vi "TIFF Default Strip Size.vi"(8 "error in (no error)":errorcluster, 10 "para1":cluster{}, 11 "para0":cluster{}) -> (0 "error out":errorcluster, 2 "function return":u32, 3 "para0 out":cluster{})   [LabVIEW 2018]
doc: "LIBTIFF_DLL_IMPEXP uint32 TIFFDefaultStripSize(TIFF*, uint32);\nextern uint32 TIFFDefaultStripSize(TIFF*, uint32);"
uses:
  libtiff3.dll
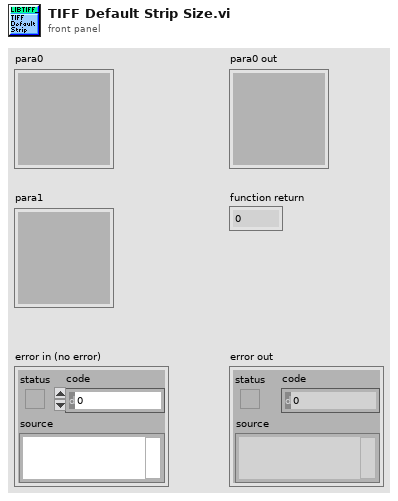
[diagram p1: front panel]
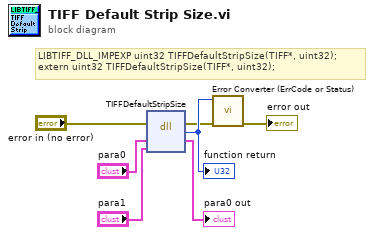
[diagram p0: block diagram]
diagram:
  # "LIBTIFF_DLL_IMPEXP\tuint32 TIFFDefaultStripSize(TIFF*, uint32);\nextern\tuint32 TIFFDefaultStripSize(TIFF*, uint32);"
  n1 = dll-call lib="C:/Users/johan/Downloads/LabVIEW software/LabVIEW software/IX-81 Software/lib/tiff/LibTiffLabview/libtiff3.*" fn="TIFFDefaultStripSize"(error in="error in (no error)", "para0"="para0", "para1"="para1") -> (error out=w2:errorcluster, w7:u32, "para0"=→"para0 out":cluster{})  [unwired: 3 in, 1 out]
  "function return" <- w7
  n2 = call "Error Converter (ErrCode or Status).vi"("error in (no error)"=w2, "error code"=w7) -> ("error out"=→"error out":errorcluster)  [unwired: 9 in]
